vi "Sound Studio.vi"() -> ()   [LabVIEW 2014]
panel:
  in  "?":enum32{"Recording", "Mixing", "Playback"}(tab)
  in  "?":bool
  out "Recorded Signal":dynamicdata(graph)
  in  "file path (use dialog)":path
  in  "Seconds to Record":dbl
  out "Mixed Track":waveform(dbl)(graph)
  out "Track 2":waveform(dbl)(graph)
  out "Track 1":waveform(dbl)(graph)
  in  "Track 2 Volume":dbl(slide) scale=0.0..10.0
  in  "Track 1 Volume":dbl(slide) scale=0.0..10.0
  in  "Track 1":path
  in  "Track 2":path
  in  "Mixed Track File":path
  out "Waveform Graph":waveform(dbl)[](graph)
  in  "Volume":dbl(slide) scale=0.0..10.0
  in  "file path (dialog if empty)":path
  in  "?":bool
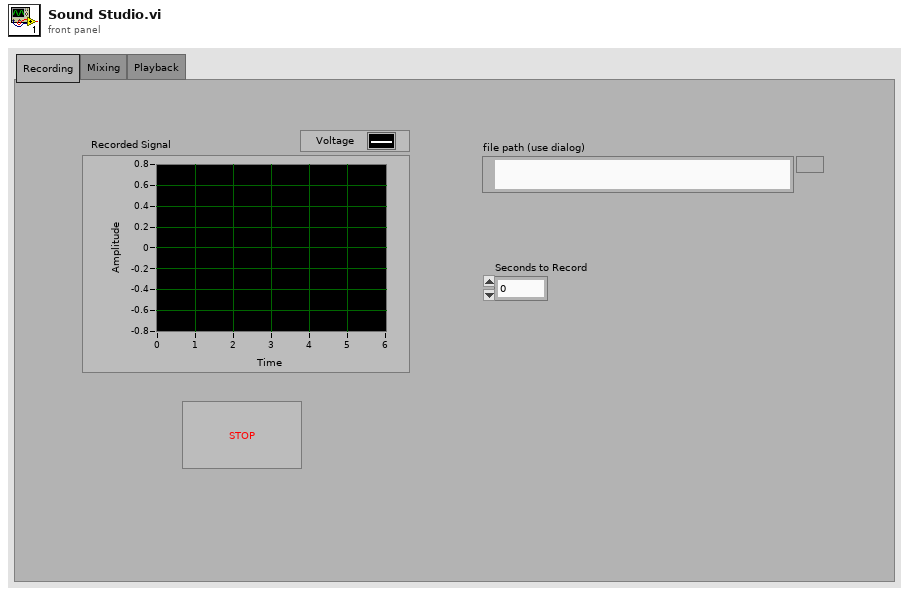
[diagram p1: front panel]
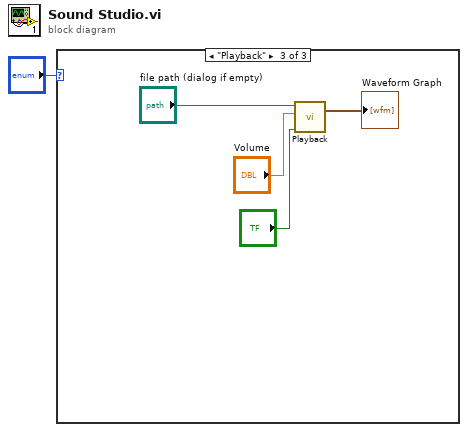
[diagram p0: block diagram]
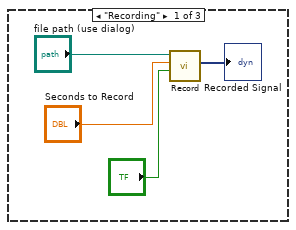
[diagram p2: hidden frame]
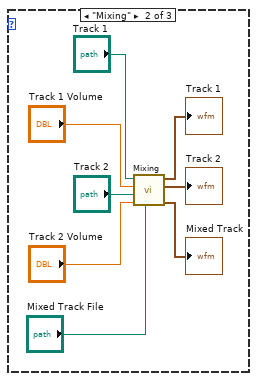
[diagram p3: hidden frame]
diagram:
  n1 = case shown="\"Playback\"" "?" {
    frame "Recording" {
      n2 = call "Record.vi"("stop (F)"="?", "Seconds to Record"="Seconds to Record", "file path (dialog if empty)"="file path (use dialog)") -> ("Recorded Signal"=→"Recorded Signal":dynamicdata)  [unwired: 8 in]
    }
    frame "Mixing" {
      n3 = call "Mixing.vi"("Mixed Track"="Mixed Track File", "Track 2 Volume"="Track 2 Volume", "Track 2"="Track 2", "Track 1 Volume"="Track 1 Volume", "Track 1"="Track 1") -> ("Mixed Track"=→"Mixed Track":waveform(dbl), "Track 2"=→"Track 2":waveform(dbl), "Track 1"=→"Track 1":waveform(dbl))  [unwired: 4 in]
    }
    frame "Playback" {
      n4 = call "Playback.vi"("stop"="?", "Volume"="Volume", "file path (dialog if empty)"="file path (dialog if empty)") -> ("Waveform Graph"=→"Waveform Graph":waveform(dbl)[])  [unwired: 8 in]
    }
  }
